vi "Start Sync.vi"(8 "error in (no error)":errorcluster, 11 "gRPC Server in":refnum<class "Query Server.lvclass">) -> (0 "error out":errorcluster, 3 "gRPC Server out":refnum<class "Query Server.lvclass">)   [LabVIEW 2016, in "Query Server.lvlib" / "Query Server.lvclass"]
uses:
  Query Server.lvclass
  gRPC lvSupport/Server API/typeDefs/grpcId.ctl
  gRPC lvSupport/gprc-lvsupport.lvlib
  RPC Messages/ServerEvent/ServerEvent_Data.ctl
  RPC Messages/QueryResponse/QueryResponse_Data.ctl
  RPC Messages/InvokeResponse/InvokeResponse_Data.ctl
panel:
  in  "Table Control":string[][](table)
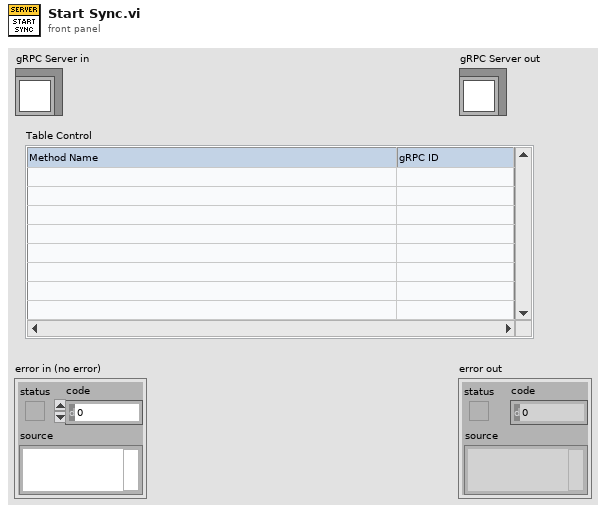
[diagram p1: front panel]
types:
  T1 = typedef "Query Server.lvlib/gprc-lvsupport.lvlib/grpcId.ctl" = u64
  T2 = typedef "Query Server.lvlib/Query Server.lvclass/ServerEvent_Data.ctl" = cluster{"eventData":string, "serverId":i32, "status":i32}
  T3 = typedef "Query Server.lvlib/Query Server.lvclass/QueryResponse_Data.ctl" = cluster{"message":string, "status":i32}
  T4 = typedef "Query Server.lvlib/Query Server.lvclass/InvokeResponse_Data.ctl" = cluster{"status":i32}
  T5 = typedef "Query Server.lvlib/Query Server.lvclass/Server gRPC UEs.ctl" = cluster{"Invoke gRPC UE":refnum<user-event>, "Query gRPC UE":refnum<user-event>, "Register gRPC UE":refnum<user-event>}
  T6 = typedef "Query Server.lvlib/Query Server.lvclass/RegistrationRequest_Data.ctl" = cluster{"eventName":string}
  T7 = typedef "Query Server.lvlib/Query Server.lvclass/QueryRequest_Data.ctl" = cluster{"query":string}
  T8 = typedef "Query Server.lvlib/Query Server.lvclass/InvokeRequest_Data.ctl" = cluster{"command":string, "parameter":string}
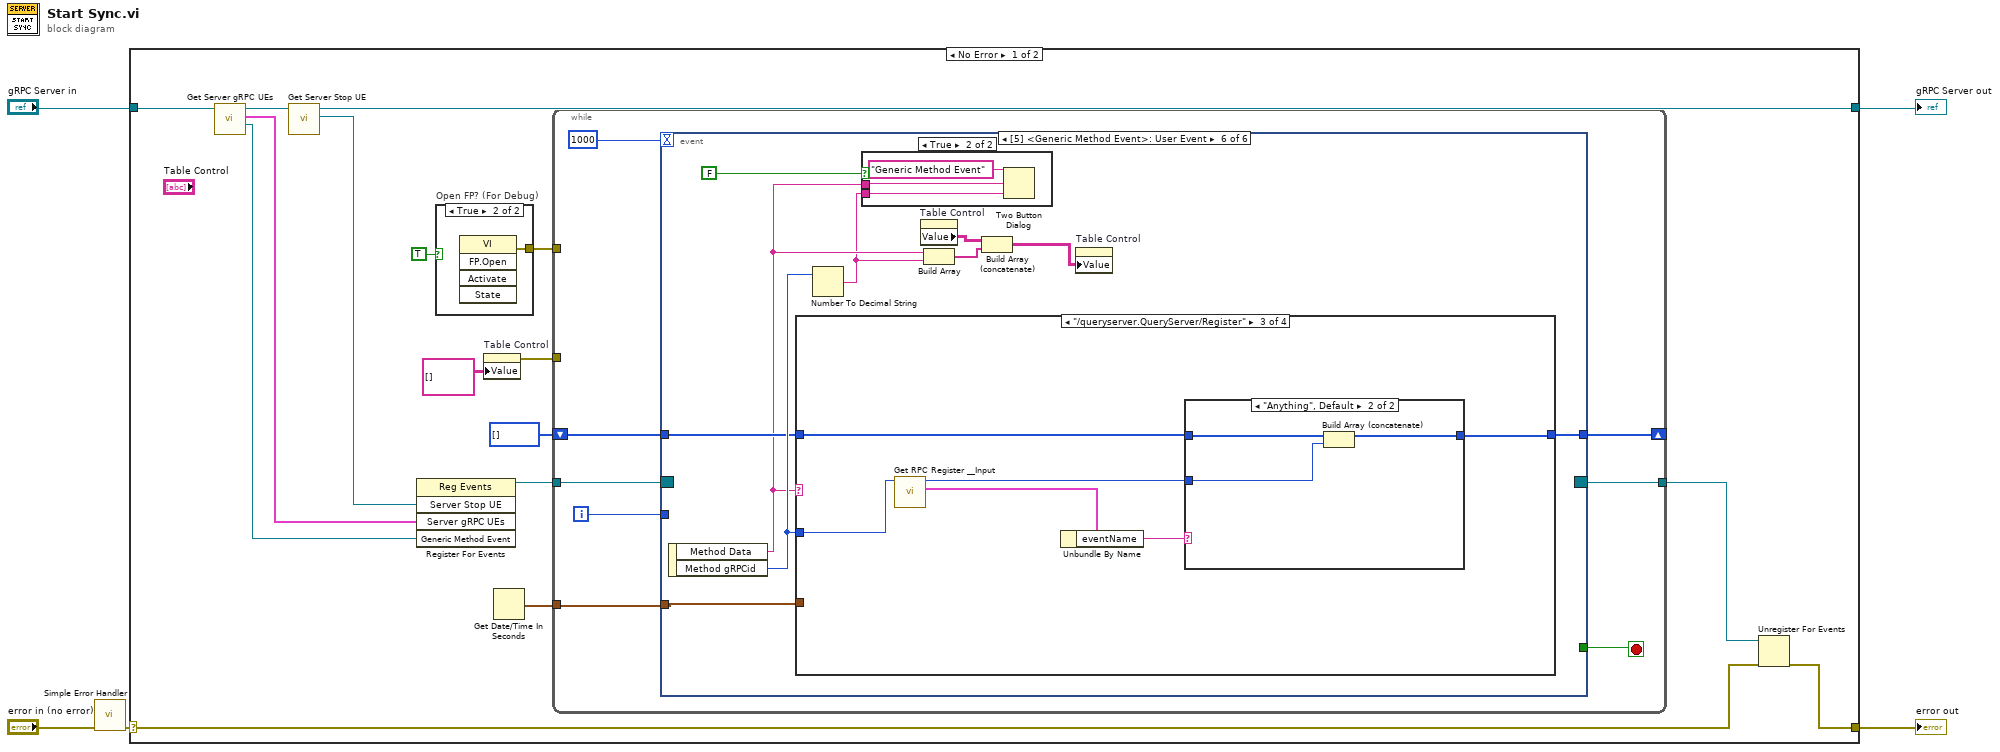
[diagram p0: block diagram]
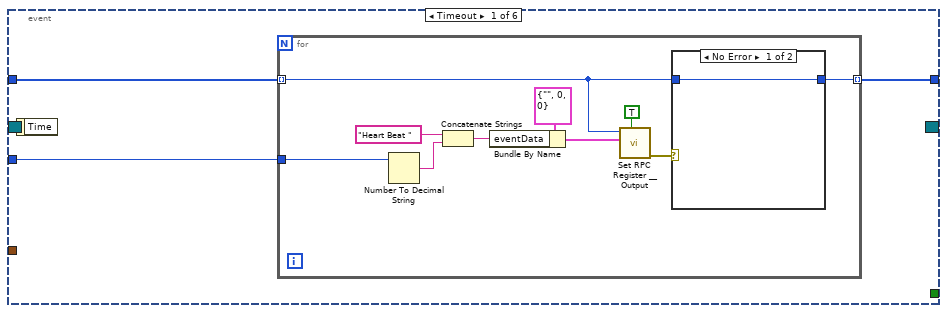
[diagram p3: hidden frame]
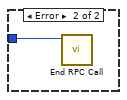
[diagram p4: hidden frame]
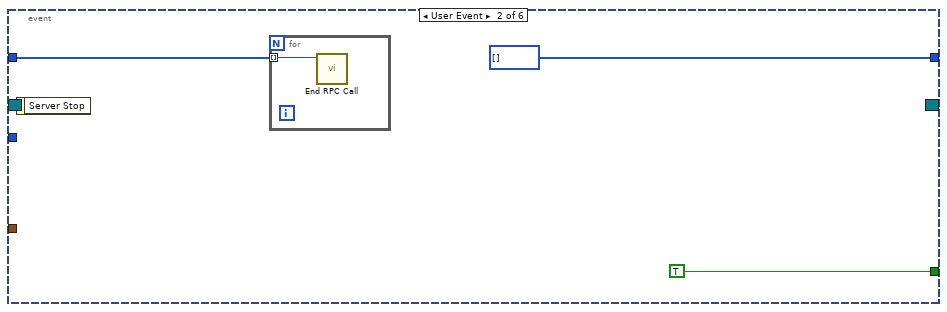
[diagram p5: hidden frame]
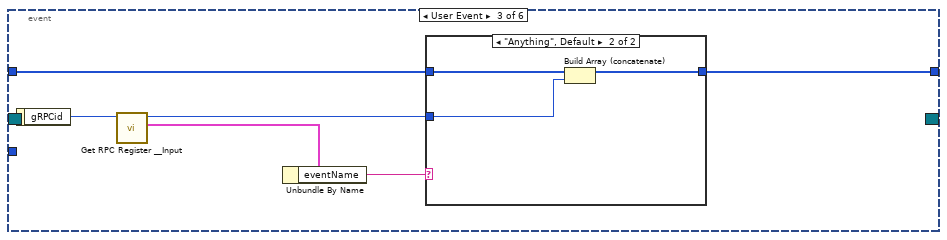
[diagram p6: hidden frame]
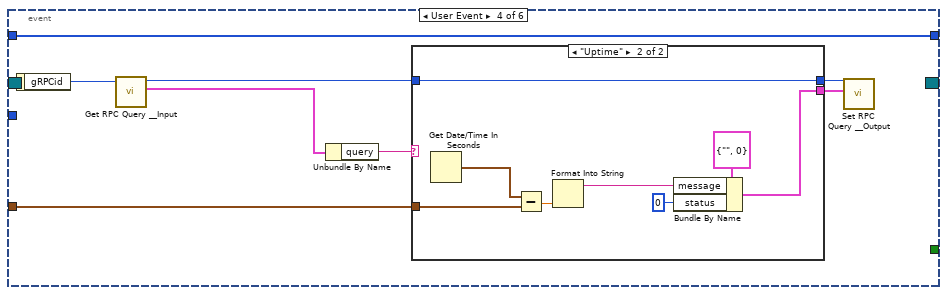
[diagram p8: hidden frame]
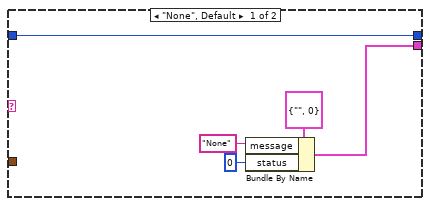
[diagram p9: hidden frame]
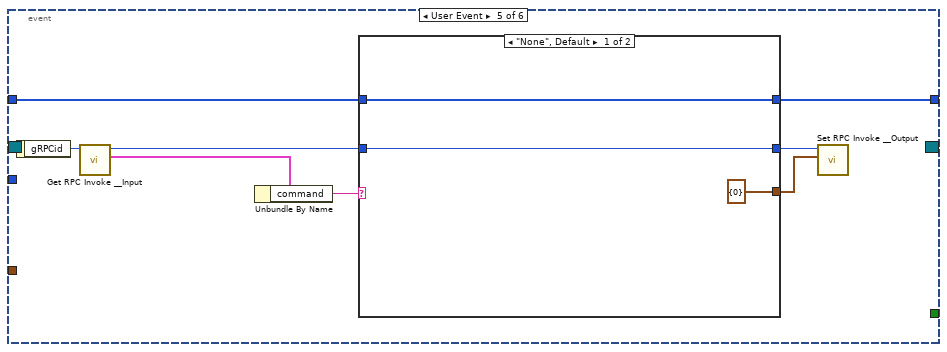
[diagram p10: hidden frame]
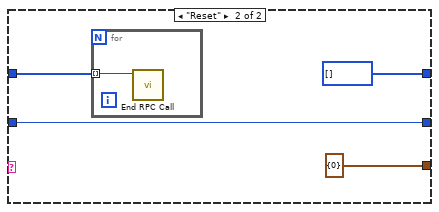
[diagram p11: hidden frame]
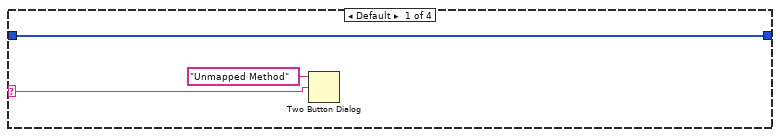
[diagram p12: hidden frame]
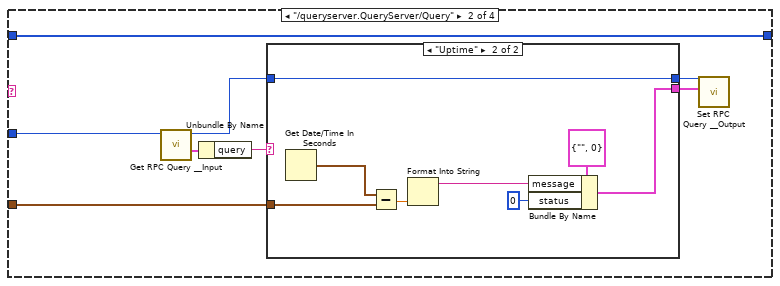
[diagram p13: hidden frame]
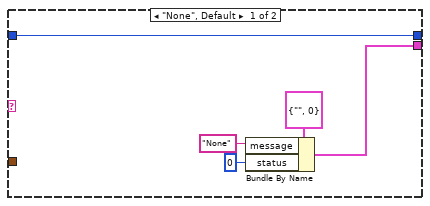
[diagram p14: hidden frame]
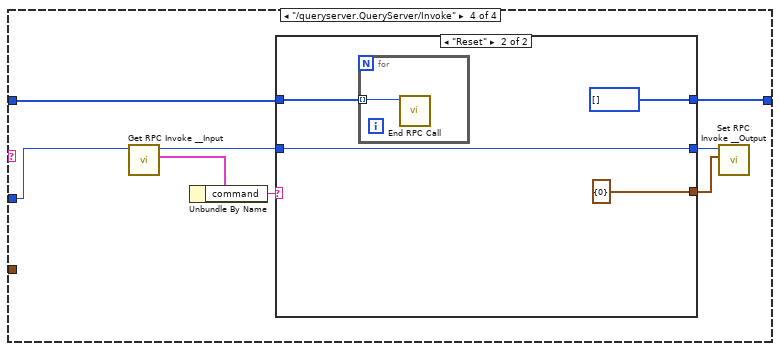
[diagram p16: hidden frame]
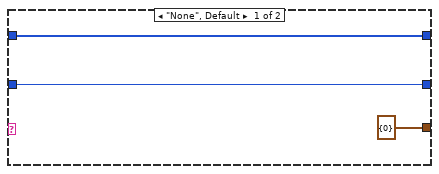
[diagram p17: hidden frame]
diagram:
  n1 = call <vilib>:"Simple Error Handler.vi"("error in (no error)"="error in (no error)") -> ("error out"=w1:errorcluster)  [unwired: 4 in, 4 out]
  n2 = case shown="No Error" w1 {
    selector: w1 -> [w14 w161]
    tunnel: [w13 w161] -> w4
    tunnel: [w17 w160] -> w2
    tunnel: "gRPC Server in" -> [w21 w160]
    frame No Error {
      n3 = call "Get Server gRPC UEs.vi"("OOP Server in"=w21) -> ("Generic Method Event"=w10:refnum<user-event>, "Server gRPC UEs"=w18:T5, "OOP Server out"=w20:refnum<class "Query Server.lvclass">)  [unwired: 8 in]
      n4 = call "Get Server Stop UE.vi"("OOP Server in"=w20) -> ("Server Stop UE"=w19:refnum<user-event>, "OOP Server out"=w17:refnum<class "Query Server.lvclass">)  [unwired: 9 in]
      n5 = register-events(w19, w18, w10) -> (reference out=w16:refnum<event-registration>)  [unwired: 2 in, 1 out]
      n6 = case "Open FP? (For Debug)" shown="True" TRUE {
        tunnel: [_ w22] -> w7
        frame False {
        }
        frame True {
          n7 = invoke class="VI" method="FP.Open"() -> (error out=w22:errorcluster)  [unwired: 5 in, 4 out]
        }
      }
      n8 = property on="Table Control" class="Tbl (strict)"("Value"=string[][] [] ("Table Control")) -> (error out=w9:errorcluster)  [unwired: 2 in, 1 out]
      n9 = Get Date/Time In Seconds() -> (seconds since 1Jan1904=w12:timestamp)
      n10 = while {
        tunnel: w16 -> [w30]
        tunnel: [w28] -> w15
        shift-right: [w26] -> _
        shift-left: T1[] [] -> [w25]
        tunnel: w12 -> [w23]
        tunnel: w9 -> [_]
        tunnel: w7 -> [_]
        i -> [w24]
        stop <- w29 stop-if-true
        n11 = event "RPC Methods Event Structure" shown="[5] <Generic Method Event>: User Event" {
          selector: w30 -> [_ _ _ _ _ _]
          dyn-events: [_ _ _ _ _ _] -> w28
          timeout: 1000 -> [_ _ _ _ _ _]
          tunnel: [_ TRUE _ _ _ _] -> w29
          tunnel: [w31 T1[] [] w51 w67 w81 w103] -> w26
          tunnel: w25 -> [w33 w47 w50 w67 w88 w102]
          tunnel: w24 -> [w32 _ _ _ _ _]
          tunnel: w23 -> [_ _ _ w61 _ w106]
          event Timeout {
            n12 = event-data() -> ()  [unwired: 1 in, 1 out]
            n13 = for {
              tunnel: w33 -> [w37] mode=indexing
              tunnel: w32 -> [w38]
              tunnel: [w35] -> w31 mode=indexing
              n14 = Number To Decimal String(number=w38) -> (decimal integer string=w43:string)  [unwired: 1 in]
              n15 = Concatenate Strings("Heart Beat " ("eventdata"), w43) -> (w41:string)
              n16 = Bundle By Name(cluster=T2 {"eventData"="", "serverId"=0, "status"=0} ("Message Data"), "eventData"=w41) -> (w39:T2)
              n17 = call "Set RPC Register __Output.vi"("Streeming? (F)"=TRUE, "Message Data"=w39, "gRPCid in"=w37) -> ("error out"=w36:errorcluster)  [unwired: 8 in]
              n18 = case shown="No Error" w36 {
                tunnel: w37 -> [w44 w45]
                tunnel: [w44 _] -> w35
                frame No Error {
                }
                frame Error {
                  n19 = call "End RPC Call.vi"("gRPCid"=w45) -> ()  [unwired: 10 in, 1 out]
                }
              }
            }
          }
          event User Event {
            n20 = event-data() -> ()  [unwired: 1 in, 1 out]
            n21 = for {
              tunnel: w47 -> [w49] mode=indexing
              n22 = call "End RPC Call.vi"("gRPCid"=w49) -> ()  [unwired: 10 in, 1 out]
            }
          }
          event User Event {
            n23 = event-data() -> ("gRPCid"=w55:T1)  [unwired: 1 in]
            n24 = call "Get RPC Register __Input.vi"("gRPCid in"=w55) -> ("Message Data"=w54:T6, "gRPCid out"=w52:T1)  [unwired: 8 in, 1 out]
            n25 = Unbundle By Name(w54) -> ("eventName"=w53:string)
            n26 = case shown="\"Anything\", Default" w53 {
              tunnel: w52 -> [_ w59]
              tunnel: [w56 w58] -> w51
              tunnel: w50 -> [w56 w57]
              frame "None" {
              }
              frame "Anything", Default {
                n27 = Build Array (concatenate)(w57, w59) -> (w58:T1[])
              }
            }
          }
          event User Event {
            n28 = event-data() -> ("gRPCid"=w66:T1)  [unwired: 1 in]
            n29 = call "Get RPC Query __Input.vi"("gRPCid in"=w66) -> ("Message Data"=w65:T7, "gRPCid out"=w63:T1)  [unwired: 8 in, 1 out]
            n30 = Unbundle By Name(w65) -> ("query"=w64:string)
            n31 = case shown="\"Uptime\"" w64 {
              tunnel: w63 -> [w72 w80]
              tunnel: [w72 w80] -> w62
              tunnel: w61 -> [_ w75]
              tunnel: [w69 w73] -> w60
              frame "None", Default {
                n32 = Bundle By Name(cluster=T3 {"message"="", "status"=0} ("Message Data"), "message"="None", "status"=0) -> (w69:T3)
              }
              frame "Uptime" {
                n33 = Get Date/Time In Seconds() -> (seconds since 1Jan1904=w79:timestamp)
                n34 = Subtract(x=w79, y=w75) -> (x-y=w78:dbl)
                n35 = Format Into String(w78) -> (resulting string=w77:string)  [unwired: 3 in, 1 out]
                n36 = Bundle By Name(cluster=T3 {"message"="", "status"=0} ("Message Data"), "message"=w77, "status"=0) -> (w73:T3)
              }
            }
            n37 = call "Set RPC Query __Output.vi"("Message Data"=w60, "gRPCid in"=w62) -> ()  [unwired: 9 in, 1 out]
          }
          event User Event {
            n38 = event-data() -> ("gRPCid"=w87:T1)  [unwired: 1 in]
            n39 = call "Get RPC Invoke __Input.vi"("gRPCid in"=w87) -> ("Message Data"=w86:T8, "gRPCid out"=w84:T1)  [unwired: 8 in, 1 out]
            n40 = Unbundle By Name(w86) -> ("command"=w85:string)
            n41 = case shown="\"None\", Default" w85 {
              tunnel: w88 -> [w91 w93]
              tunnel: w84 -> [w90 w95]
              tunnel: [w90 w95] -> w83
              tunnel: [T4 {"status"=0} ("Message Data") T4 {"status"=0} ("Message Data")] -> w82
              tunnel: [w91 T1[] []] -> w81
              frame "None", Default {
              }
              frame "Reset" {
                n42 = for {
                  tunnel: w93 -> [w96] mode=indexing
                  n43 = call "End RPC Call.vi"("gRPCid"=w96) -> ()  [unwired: 10 in, 1 out]
                }
              }
            }
            n44 = call "Set RPC Invoke __Output.vi"("Message Data"=w82, "gRPCid in"=w83) -> ()  [unwired: 9 in, 1 out]
          }
          event User Event {
            n45 = event-data() -> ("Method Data"=w101:string, "Method gRPCid"=w105:T1)  [unwired: 1 in]
            n46 = case shown="\"/queryserver.QueryServer/Register\"" w101 {
              selector: w101 -> [w107 _ _ _]
              tunnel: w106 -> [_ w112 _ _]
              tunnel: w105 -> [_ w111 w131 w141]
              tunnel: [w109 w110 w132 w142] -> w103
              tunnel: w102 -> [w109 w110 w133 w143]
              frame Default {
                n47 = Two Button Dialog(message="Unmapped Method", 2:w107) -> ()  [unwired: 1 in, 1 out]
              }
              frame "/queryserver.QueryServer/Query" {
                n48 = call "Get RPC Query __Input.vi"("gRPCid in"=w111) -> ("Message Data"=w117:T7, "gRPCid out"=w115:T1)  [unwired: 8 in, 1 out]
                n49 = Unbundle By Name(w117) -> ("query"=w116:string)
                n50 = case shown="\"Uptime\"" w116 {
                  tunnel: w115 -> [w122 w130]
                  tunnel: [w122 w130] -> w114
                  tunnel: w112 -> [_ w125]
                  tunnel: [w119 w123] -> w113
                  frame "None", Default {
                    n51 = Bundle By Name(cluster=T3 {"message"="", "status"=0} ("Message Data"), "message"="None", "status"=0) -> (w119:T3)
                  }
                  frame "Uptime" {
                    n52 = Get Date/Time In Seconds() -> (seconds since 1Jan1904=w129:timestamp)
                    n53 = Subtract(x=w129, y=w125) -> (x-y=w128:dbl)
                    n54 = Format Into String(w128) -> (resulting string=w127:string)  [unwired: 3 in, 1 out]
                    n55 = Bundle By Name(cluster=T3 {"message"="", "status"=0} ("Message Data"), "message"=w127, "status"=0) -> (w123:T3)
                  }
                }
                n56 = call "Set RPC Query __Output.vi"("Message Data"=w113, "gRPCid in"=w114) -> ()  [unwired: 9 in, 1 out]
              }
              frame "/queryserver.QueryServer/Register" {
                n57 = call "Get RPC Register __Input.vi"("gRPCid in"=w131) -> ("Message Data"=w136:T6, "gRPCid out"=w134:T1)  [unwired: 8 in, 1 out]
                n58 = Unbundle By Name(w136) -> ("eventName"=w135:string)
                n59 = case shown="\"Anything\", Default" w135 {
                  tunnel: w134 -> [_ w140]
                  tunnel: [w137 w139] -> w132
                  tunnel: w133 -> [w137 w138]
                  frame "None" {
                  }
                  frame "Anything", Default {
                    n60 = Build Array (concatenate)(w138, w140) -> (w139:T1[])
                  }
                }
              }
              frame "/queryserver.QueryServer/Invoke" {
                n61 = call "Get RPC Invoke __Input.vi"("gRPCid in"=w141) -> ("Message Data"=w148:T8, "gRPCid out"=w146:T1)  [unwired: 8 in, 1 out]
                n62 = Unbundle By Name(w148) -> ("command"=w147:string)
                n63 = case shown="\"Reset\"" w147 {
                  tunnel: w143 -> [w151 w153]
                  tunnel: w146 -> [w150 w155]
                  tunnel: [w150 w155] -> w145
                  tunnel: [T4 {"status"=0} ("Message Data") T4 {"status"=0} ("Message Data")] -> w144
                  tunnel: [w151 T1[] []] -> w142
                  frame "None", Default {
                  }
                  frame "Reset" {
                    n64 = for {
                      tunnel: w153 -> [w156] mode=indexing
                      n65 = call "End RPC Call.vi"("gRPCid"=w156) -> ()  [unwired: 10 in, 1 out]
                    }
                  }
                }
                n66 = call "Set RPC Invoke __Output.vi"("Message Data"=w144, "gRPCid in"=w145) -> ()  [unwired: 9 in, 1 out]
              }
            }
            n67 = Number To Decimal String(number=w105) -> (decimal integer string=w100:string)  [unwired: 1 in]
            n68 = case shown="True" FALSE {
              tunnel: w101 -> [_ w158]
              tunnel: w100 -> [_ w157]
              frame False {
              }
              frame True {
                n69 = Two Button Dialog(message="Generic Method Event", 1:w157, 2:w158) -> ()  [unwired: 1 out]
              }
            }
            n70 = property on="Table Control" class="Tbl (strict)"() -> ("Value"=w99:string[][])  [unwired: 2 in, 2 out]
            n71 = Build Array(w101, w100) -> (w98:string[])
            n72 = Build Array (concatenate)(w99, w98) -> (w97:string[][])
            n73 = property on="Table Control" class="Tbl (strict)"("Value"=w97) -> ()  [unwired: 2 in, 2 out]
          }
        }
      }
      n74 = Unregister For Events(event registration refnum=w15, error in=w14) -> (error out=w13:errorcluster)
    }
    frame Error {
    }
  }
  "error out" <- w4
  "gRPC Server out" <- w2
